vi "Registered PV to Typedescriptor.vi"(8 "Error In":errorcluster, 11 "Registered PV":T1) -> (0 "Error Out":errorcluster, 3 "Type Descriptor":string)   [LabVIEW 2015, in "CS++DIMMonitor.lvlib" / "CS++DIMMonitor.lvclass"]
doc: "Read PV type descriptor from registered PV command."
uses:
  CS++DIMMonitor.lvclass
  <vilib>/ActorFramework/Message Enqueuer/Message Enqueuer.lvclass
  CSPP_Core/Actors/CS++PVMonitor Messages/CS++PVUpdate Msg/CS++PVUpdate Msg.lvclass
  CSPP_Core/Actors/CS++PVMonitor Messages/CS++PVUpdate Msg/CS++PVUpdate Msg.lvclass/CS++PVUpdate Msg.ctl
  CSPP_Core/Classes/CS++ProcessVariables/ProcessVariable/PV.lvclass/PV.ctl
  CSPP_Core/Classes/CS++ProcessVariables/ProcessVariable/PV.lvclass
  DIMConnection/DIMConnection.lvclass
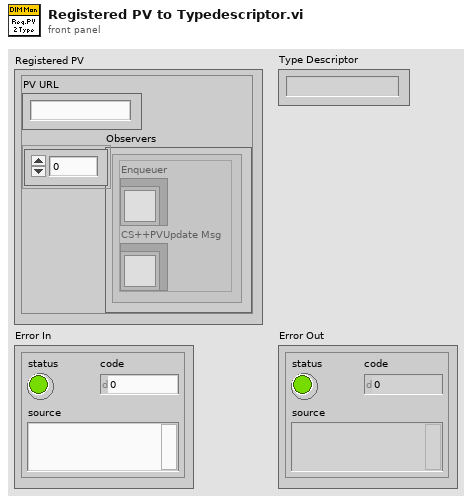
[diagram p1: front panel]
types:
  T1 = cluster{"PV URL":string, "Observers":cluster{"Enqueuer":refnum<class "Message Enqueuer.lvclass">, "CS++PVUpdate Msg":refnum<class "CS++PVUpdate Msg.lvclass">}[]}
  T2 = cluster{"Enqueuer":refnum<class "Message Enqueuer.lvclass">, "CS++PVUpdate Msg":refnum<class "CS++PVUpdate Msg.lvclass">}[]
  T3 = cluster{"Enqueuer":refnum<class "Message Enqueuer.lvclass">, "CS++PVUpdate Msg":refnum<class "CS++PVUpdate Msg.lvclass">}
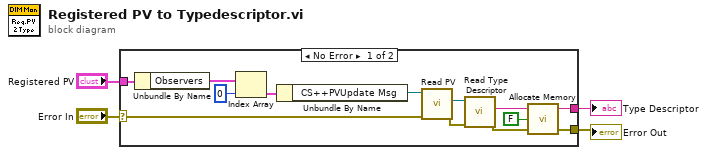
[diagram p0: block diagram]
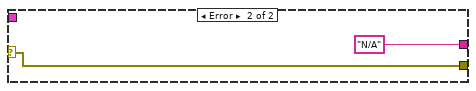
[diagram p2: hidden frame]
diagram:
  n1 = case shown="No Error" "Error In" {
    selector: "Error In" -> [w10 w19]
    tunnel: "Registered PV" -> [w14 _]
    tunnel: [w6 w19] -> w2
    tunnel: [w8 "N/A" ("Type Descriptor")] -> w1
    frame No Error {
      n2 = Unbundle By Name(w14) -> ("Observers"=w17:T2)
      n3 = Index Array(array=w17, index=0) -> (element=w15:T3)
      n4 = Unbundle By Name(w15) -> ("CS++PVUpdate Msg"=w13:refnum<class "CS++PVUpdate Msg.lvclass">)
      n5 = call "Read PV.vi"("error in (no error)"=w10, "CS++PVUpdate Msg in"=w13) -> ("error out"=w11:errorcluster, "PV"=w12:refnum<class "PV.lvclass">)  [unwired: 7 in, 1 out]
      n6 = call "Read Type Descriptor.vi"("error in (no error)"=w11, "PV in"=w12) -> ("error out"=w7:errorcluster, "Type Descriptor"=w9:string)  [unwired: 7 in, 1 out]
      n7 = call "Allocate Memory.vi"("Error In"=w7, "Allocate Memory? (T)"=FALSE, "Type Descriptor"=w9) -> ("Error Out"=w6:errorcluster, "dup Type Descriptor"=w8:string)  [unwired: 1 out]
    }
    frame Error {
    }
  }
  "Error Out" <- w2
  "Type Descriptor" <- w1
